vi "Read Filter status.vi"(8 "error in (no error)":errorcluster, 11 "Filter params in":refnum<class "CV-Filter.lvclass">) -> (0 "error out":errorcluster, 2 "Acquisition status":T1, 3 "Filter params out":refnum<class "CV-Filter.lvclass">)   [LabVIEW 2013, in "CameraVision.lvlib" / "CV-Filter.lvclass"]
uses:
  CV-Filter.lvclass
  UI/Module-states.ctl
  CV-Filter.lvclass/CV-Filter.ctl
  UI/CV-UI.lvclass
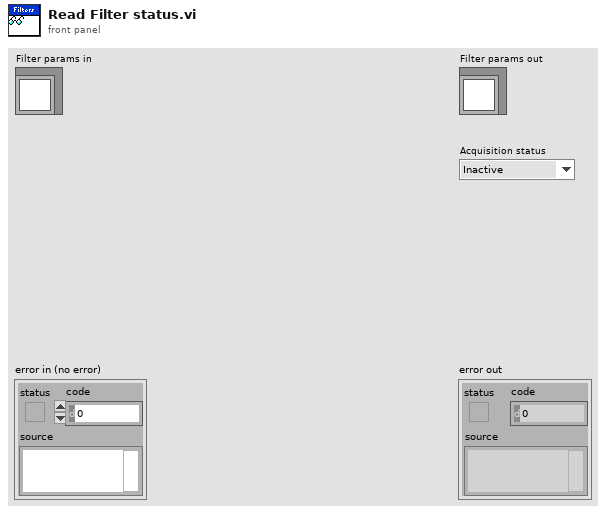
[diagram p1: front panel]
types:
  T1 = typedef "CameraVision.lvlib/CV-UI.lvclass/Module-states.ctl" = enum16{"Inactive", "Active", "Data-loss", "Error", "Simulation", "Synchronizing", "Initialized", "Released"}
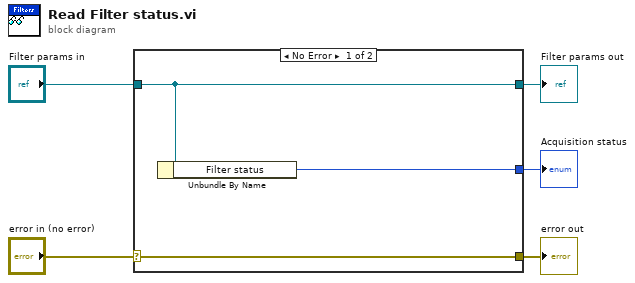
[diagram p0: block diagram]
diagram:
  n1 = case shown="No Error" "error in (no error)" {
    selector: "error in (no error)" -> [w8 w9]
    tunnel: [w8 w9] -> w4
    tunnel: [w7 w10] -> w2
    tunnel: "Filter params in" -> [w7 w10]
    tunnel: [w6 _] -> w1
    frame No Error {
      n2 = Unbundle By Name(w7) -> ("Filter status"=w6:T1)
    }
    frame Error {
    }
  }
  "error out" <- w4
  "Filter params out" <- w2
  "Acquisition status" <- w1
